vi "IBM4_Diff_Read(V1).vi"(8 "error in":errorcluster, 9 "Neg-Chan":i32=1, 10 "Pos-Chan":i32, 11 "COM resource in":refnum<visa-resource-name>="COM9") -> (0 "error out":errorcluster, 2 "output":dbl, 3 "COM resource out":refnum<visa-resource-name>)   [LabVIEW 2022 SP3, in "IBM4.lvlib"]
doc: "This VI interfaces with the IBM4 to perform a differential read operation.\n\nThe input channels must be between 0 and 4, while the output will be in floating point format (thus, in Volts).\nOnly a single read operation is made with this VI. \n\nAlternate read operations exist covering binary or floating point, single reading, multiple readings, and an average of multiple readings (floating point only)."
uses:
  <instrlib>/IBM4/IBM4.lvlib
panel:
  out "error out 2":errorcluster
  out "read buffer":string
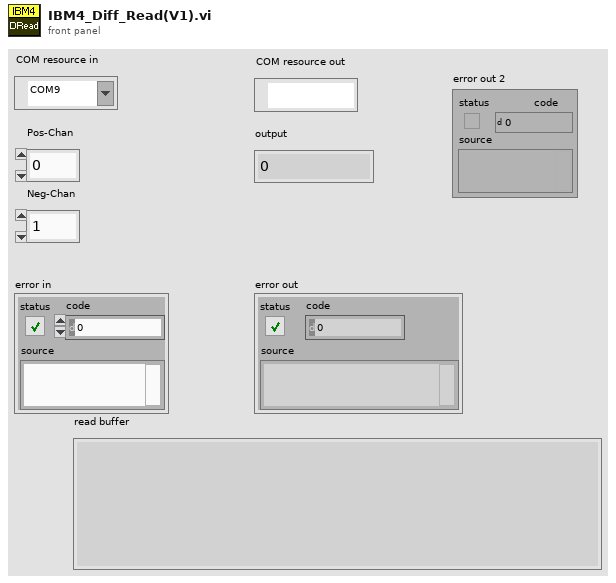
[diagram p1: front panel]
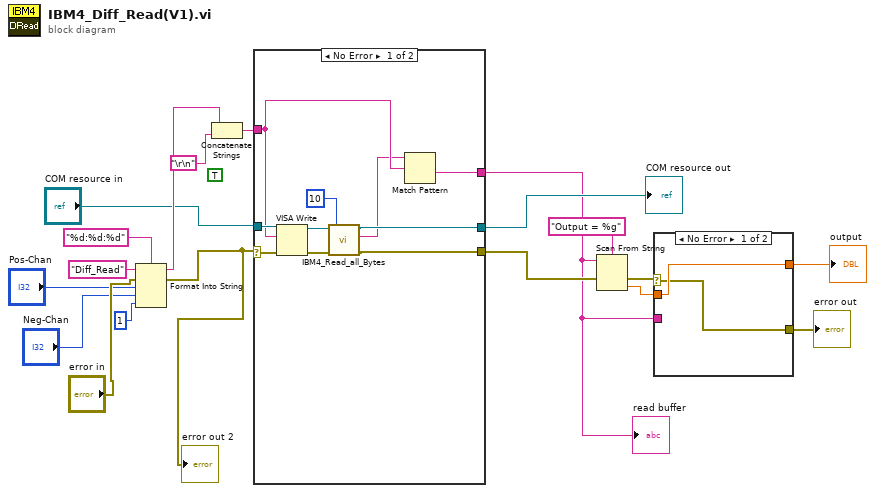
[diagram p0: block diagram]
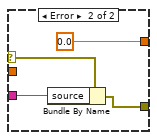
[diagram p2: hidden frame]
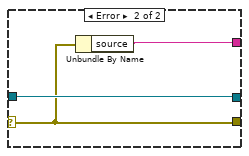
[diagram p3: hidden frame]
diagram:
  (unwired) TRUE ("Enable Termination\nChar (T)")
  n1 = Format Into String(format string="%d:%d:%d", initial string="Diff_Read", error in="error in", "Pos-Chan", "Neg-Chan", 1 ("input 2")) -> (resulting string=w11:string, error out=w1:errorcluster)
  "error out 2" <- w1
  n2 = Concatenate Strings(w11, "\r\n") -> (w10:string)
  n3 = case shown="No Error" w1 {
    selector: w1 -> [w26 w30]
    tunnel: "COM resource in" -> [w29 w32]
    tunnel: [w21 w30] -> w14
    tunnel: [w28 w31] -> w6
    tunnel: w10 -> [w27 _]
    tunnel: [w22 w32] -> w15
    frame No Error {
      n4 = VISA Write(VISA resource name=w29, write buffer=w27, error in (no error)=w26) -> (VISA resource name out=w25:refnum<visa-resource-name>, error out=w24:errorcluster)  [unwired: 1 out]
      n5 = call <instrlib>:"IBM4_Read_all_Bytes.vi"("error in (no error)"=w24, "milliseconds to wait"=u32 10, "VISA Refnum in"=w25) -> ("error out"=w21:errorcluster, "String"=w20:string, "VISA Refnum out"=w22:refnum<visa-resource-name>)  [unwired: 2 in]
      n6 = Match Pattern(string=w20, regular expression=w27) -> (after substring=w28:string)  [unwired: 1 in, 3 out]
    }
    frame Error {
      n7 = Unbundle By Name(w30) -> ("source"=w31:string)
    }
  }
  "COM resource out" <- w15
  "read buffer" <- w6
  n8 = Scan From String(format string="Output = %g", input string=w6, error in=w14) -> (error out=w9:errorcluster, output 1=w3:dbl)  [unwired: 2 in, 2 out]
  n9 = case shown="No Error" w9 {
    selector: w9 -> [w33 w37]
    tunnel: w3 -> [w34 _]
    tunnel: [w34 0.0] -> w8
    tunnel: [w33 w35] -> w7
    tunnel: w6 -> [_ w36]
    frame No Error {
    }
    frame Error {
      n10 = Bundle By Name(cluster=w37, "source"=w36) -> (w35:errorcluster)
    }
  }
  "error out" <- w7
  "output" <- w8
